vi "LVClass_WavefrontCorrector Move Actuator to Absolute Position.vi"(0 "WavefrontCorrector in":refnum<class "WavefrontCorrector.lvclass">, 5 "Index of actuator":i32, 7 "Position":sgl, 11 "error in (no error)":errorcluster) -> (4 "WavefrontCorrector out":refnum<class "WavefrontCorrector.lvclass">, 15 "error out":errorcluster)   [LabVIEW 2020, in "WavefrontCorrector.lvclass"]
uses:
  WavefrontCorrector.lvclass
  WavefrontCorrector.lvclass/WavefrontCorrector.ctl
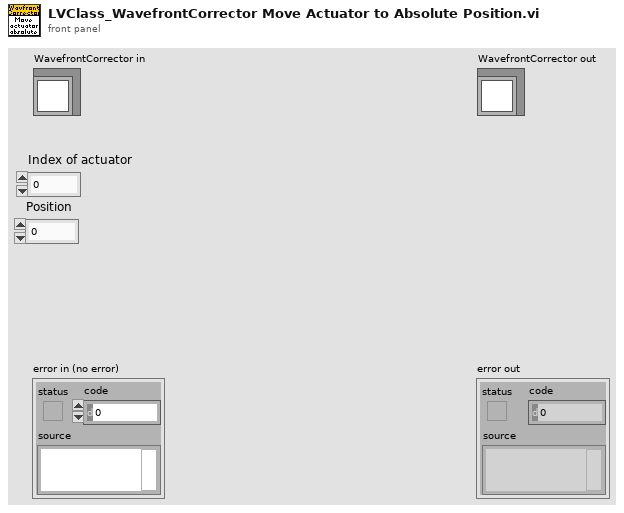
[diagram p1: front panel]
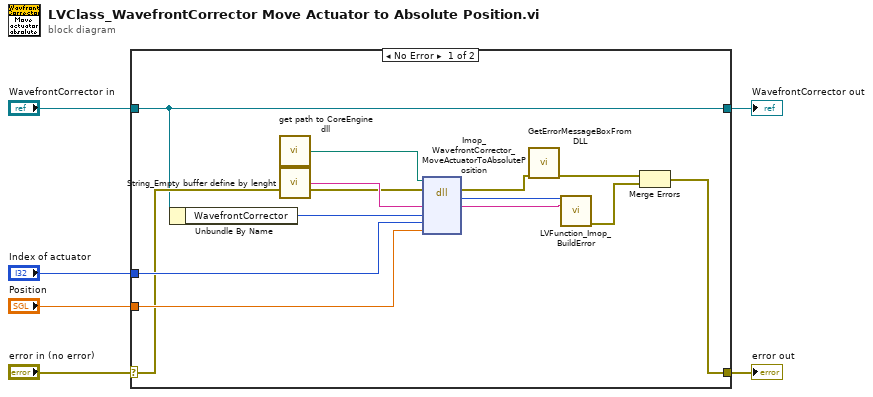
[diagram p0: block diagram]
diagram:
  n1 = case shown="No Error" "error in (no error)" {
    selector: "error in (no error)" -> [w9 w21]
    tunnel: [w10 w21] -> w5
    tunnel: [w8 w20] -> w3
    tunnel: "WavefrontCorrector in" -> [w8 w20]
    tunnel: "Index of actuator" -> [w12 _]
    tunnel: "Position" -> [w11 _]
    frame No Error {
      n2 = Unbundle By Name(w8) -> ("WavefrontCorrector"=w7:i32)
      n3 = call "get path to CoreEngine dll.vi"() -> ("path to c_interface_vc100.dll"=w13:path)  [unwired: 12 in, 3 out]
      n4 = call "String_Empty buffer define by lenght.vi"() -> ("Empty buffer"=w14:string)  [unwired: 1 in]
      n5 = dll-call lib="D:/FLE/0.Code/CoreEngine4_Suite/LV2011_interface/DLLs/c_interface_vc100.dll" fn="Imop_WavefrontCorrector_MoveActuatorToAbsolutePosition"(path in=w13, error in=w9, "Message"=w14, "WavefrontCorrector"=w7, "Index of actuator"=w12, "Position"=w11) -> (error out=w15:errorcluster, "return type"=w18:i32, "Message"=w19:string)  [unwired: 4 in, 1 out]
      n6 = call "GetErrorMessageBoxFromDLL.vi"("error IN"=w15) -> ("error OUT"=w16:errorcluster)  [unwired: 10 in]
      n7 = call "LVFunction_Imop_BuildError.vi"("code"=w18, "String to Prepend to source (\"\")"=w19) -> ("error out"=w17:errorcluster)  [unwired: 13 in]
      n8 = Merge Errors(w16, w17) -> (w10:errorcluster)
    }
    frame Error {
    }
  }
  "error out" <- w5
  "WavefrontCorrector out" <- w3
